vi "GetBuvVoltage (SubVI).vi"(0 "connection ID in":refnum<k5>, 5 "error in":errorcluster) -> (8 "Voltage":string, 14 "connection ID out":refnum<k5>, 19 "error out":errorcluster)   [LabVIEW 2013]
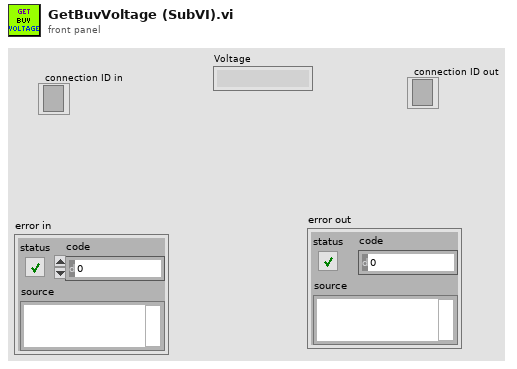
[diagram p1: front panel]
types:
  T1 = enum16{"Standard", "Buffered", "CRLF", "Immediate"}
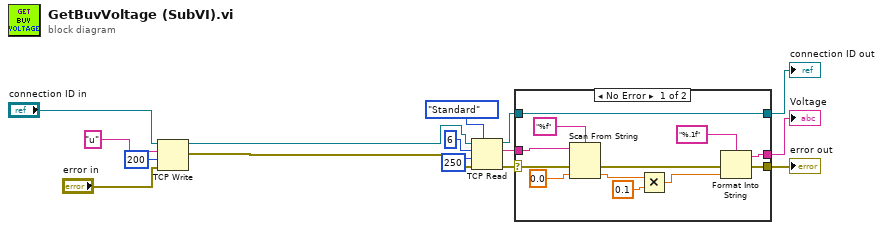
[diagram p0: block diagram]
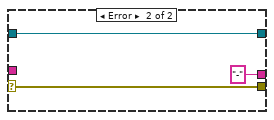
[diagram p2: hidden frame]
diagram:
  n1 = TCP Write(connection ID="connection ID in", data in="u", error in (no error)="error in", 9:200 ("timeout ms (25000)")) -> (connection ID out=w2:refnum<k5>, error out=w1:errorcluster)  [unwired: 1 out]
  n2 = TCP Read(connection ID=w2, bytes to read=6, error in (no error)=w1, 7:T1."Standard" ("mode (standard)"), 9:250 ("timeout ms (25000)")) -> (connection ID out=w7:refnum<k5>, data out=w9:string, error out=w10:errorcluster)
  n3 = case shown="No Error" w10 {
    selector: w10 -> [w18 w29]
    tunnel: [w25 "-"] -> w14
    tunnel: [w22 w29] -> w15
    tunnel: w9 -> [w17 _]
    tunnel: [w16 w28] -> w8
    tunnel: w7 -> [w16 w28]
    frame No Error {
      n4 = Scan From String(format string="%f", input string=w17, error in=w18, default 1=0.0 ("default value 1")) -> (error out=w23:errorcluster, output 1=w24:dbl)  [unwired: 1 in, 2 out]
      n5 = Multiply(x=w24, y=0.1) -> (x*y=w20:dbl)
      n6 = Format Into String(format string="%.1f", error in=w23, w20) -> (resulting string=w25:string, error out=w22:errorcluster)  [unwired: 1 in]
    }
    frame Error {
    }
  }
  "error out" <- w15
  "connection ID out" <- w8
  "Voltage" <- w14
